vi "Has Marker.vi"(8 "error in (no error)":errorcluster, 10 "Position":T1, 11 "Maze in":refnum<class "Maze.lvclass">) -> (0 "error out":errorcluster, 2 "Has Marker?":bool, 3 "Maze out":refnum<class "Maze.lvclass">)   [LabVIEW 2020, in "Maze.lvlib" / "Maze.lvclass"]
uses:
  Maze.lvclass
  Position.ctl
  Maze.lvclass/Maze.ctl
  Maze.lvlib
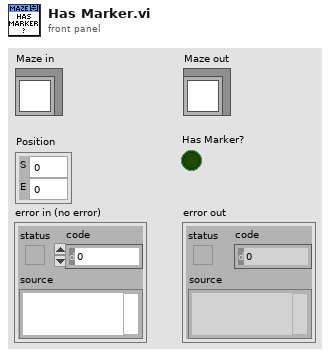
[diagram p1: front panel]
types:
  T1 = typedef "Maze.lvlib/Position.ctl" = cluster{"S":i32, "E":i32}
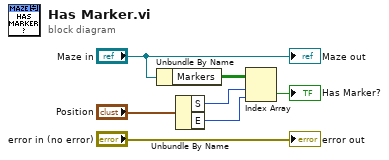
[diagram p0: block diagram]
diagram:
  n1 = Unbundle By Name("Maze in") -> ("Markers"=w5:bool[][])
  n2 = Unbundle By Name("Position") -> ("S"=w3:i32, "E"=w2:i32)
  n3 = Index Array(array=w5, index (row)=w3, index (col)=w2) -> (element=→"Has Marker?":bool)
  "error out" <- "error in (no error)"
  "Maze out" <- "Maze in"
